vi "rotate.vi"(9 "?":u8[][](array[numeric]), 11 "?":u8[][](array[numeric])) -> (3 "?":u8[][](array[numeric]))   [LabVIEW 2018]
uses:
  <vilib>/Analysis/baseanly.llb/Mean (DBL).vi
  <vilib>/Analysis/NI_AALBase.lvlib
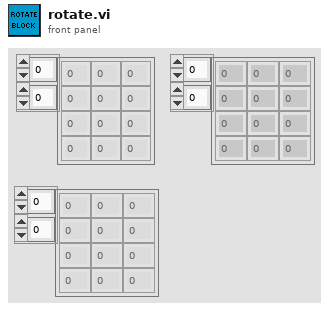
[diagram p1: front panel]
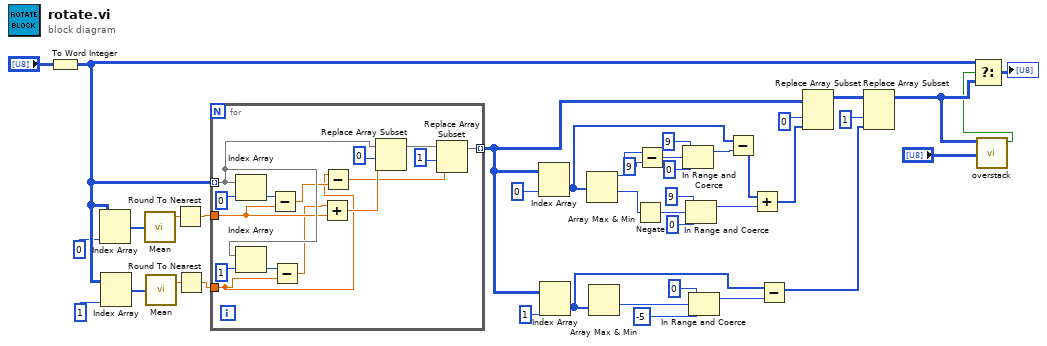
[diagram p0: block diagram]
diagram:
  n1 = To Word Integer(number="?") -> (16bit integer=w22:i16[][])
  n2 = Index Array(array=w22, index (col)=0) -> (element=w24:i16[])  [unwired: 1 in]
  n3 = Index Array(array=w22, index (col)=1) -> (element=w25:i16[])  [unwired: 1 in]
  n4 = call-poly <vilib>:"Mean.vi"("X"=w24) -> ("mean"=w27:dbl)  [unwired: 1 out]
  n5 = call-poly <vilib>:"Mean.vi"("X"=w25) -> ("mean"=w26:dbl)  [unwired: 1 out]
  n6 = Round To Nearest(number=w27) -> (nearest integer value=w28:dbl)
  n7 = Round To Nearest(number=w26) -> (nearest integer value=w29:dbl)
  n8 = for {
    tunnel: w22 -> [w53] mode=indexing
    tunnel: w28 -> [w46]
    tunnel: w29 -> [w42]
    tunnel: [w49] -> w32 mode=indexing
    n9 = Index Array(array=w53, index=0) -> (element=w48:i16)
    n10 = Index Array(array=w53, index=1) -> (element=w47:i16)
    n11 = Subtract(x=w48, y=w46) -> (x-y=w43:dbl)
    n12 = Subtract(x=w47, y=w42) -> (x-y=w45:dbl)
    n13 = Add(x=w45, y=w46) -> (x+y=w44:dbl)
    n14 = Subtract(x=w42, y=w43) -> (x-y=w41:dbl)
    n15 = Replace Array Subset(array=w53, new element=w44, index=0) -> (w50:i16[])
    n16 = Replace Array Subset(array=w50, new element=w41, index=1) -> (w49:i16[])
  }
  n17 = Index Array(array=w32, index (col)=0) -> (element=w31:i16[])  [unwired: 1 in]
  n18 = Index Array(array=w32, index (col)=1) -> (element=w37:i16[])  [unwired: 1 in]
  n19 = Array Max & Min(array=w31) -> (max value=w8:i16, min value=w15:i16)  [unwired: 2 out]
  n20 = Array Max & Min(array=w37) -> (min value=w35:i16)  [unwired: 3 out]
  n21 = Negate(x=w15) -> (-x=w16:i16)
  n22 = Subtract(x=w8, y=9) -> (x-y=w10:i32)
  n23 = In Range and Coerce(upper limit=9, x=w10, lower limit=0) -> (coerced(x)=w17:i32)  [unwired: 1 out]
  n24 = In Range and Coerce(upper limit=9, x=w16, lower limit=0) -> (coerced(x)=w18:i32)  [unwired: 1 out]
  n25 = In Range and Coerce(upper limit=0, x=w35, lower limit=-5) -> (coerced(x)=w36:i32)  [unwired: 1 out]
  n26 = Subtract(x=w31, y=w17) -> (x-y=w19:i32[])
  n27 = Add(x=w19, y=w18) -> (x+y=w21:i32[])
  n28 = Subtract(x=w37, y=w36) -> (x-y=w40:i32[])
  n29 = Replace Array Subset(array=w32, new element=w21, index (col)=0) -> (w39:i16[][])  [unwired: 1 in]
  n30 = Replace Array Subset(array=w39, new element=w40, index (col)=1) -> (w2:i16[][])  [unwired: 1 in]
  n31 = call "overstack.vi"("board array"="?", "Piece Array"=w2) -> ("Touching"=w1:bool)  [unwired: 7 in, 2 out]
  n32 = Select(t=w22, s=w1, f=w2) -> (s? t:f=→"?":i16[][])
